vi "SimpleMotion2.vi"() -> ()   [LabVIEW 2019]
uses:
  Motion/EnableMultiple.vi
  Motion/MoveIncMultiple.vi
  Motion/WaitMultiple.vi
  Motion/DisableMultiple.vi
panel:
  out "Position 2":string
  in  "Distance 2":dbl=10000.0
  in  "Speed 2":dbl=5000.0
  in  "Axis Name 2":string="Y"
  out "Position":string
  in  "Distance":dbl=10000.0
  in  "Speed":dbl=5000.0
  in  "Axis Name":string="X"
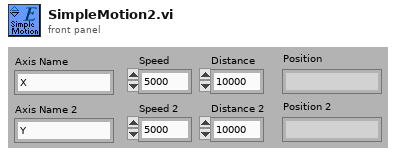
[diagram p1: front panel]
types:
  T1 = typedef "ControllerDiagPacket.ctl" = cluster{"Count":i32, "Packet Time":i64, "Axes":T2[], "error":errorcluster}
  T2 = typedef "AxisDiagPacket.ctl" = cluster{"Axis Name":string, "Acceleration Command":dbl, "Amplifier Temperature":sgl, "Analog Input 0":dbl, "Analog Input 1":dbl, "Analog Output 0":dbl, "Analog Output 1":dbl, "Axis Fault (num)":i32, "Axis Fault (str)":string, "Axis Fault (bits)":cluster{"AmplifierFault":bool, "AmplifierTemperatureFault":bool, "CcwEndOfTravelLimitFault":bool, "CcwSoftwareLimitFault":bool, "CommunicationLostFault":bool, "CwEndOfTravelLimitFault":bool, "CwSoftwareLimitFault":bool, "EmergencyStopFault":bool, "EncoderFault":bool, "ExternalFault":bool, "FeedbackScalingFault":bool, "HallSensorFault":bool, "MarkerSearchFault":bool, "MaxVelocityCommandFault":bool, "MotorTemperatureFault":bool, "None":bool, "OverCurrentFault":bool, "PositionErrorFault":bool, "PositionFeedbackFault":bool, "PowerSupplyFault":bool, "VelocityErrorFault":bool, "VelocityFeedbackFault":bool, "VoltageClampFault":bool}, "Axis Status (num)":i32, "Axis Status (str)":string, "Axis Status (bits)":cluster{"AccelerationPhase":bool, "AutofocusActive":bool, "BrakeOutput":bool, "CalibrationActive":bool, "CalibrationEnabled":bool, "CcwEndOfTravelLimitInput":bool, "CommandShapingFilterDone":bool, "CosineEncoderError":bool, "CurrentClamp":bool, "CwEndOfTravelLimitInput":bool, "DecelerationPhase":bool, "EmergencyStopInput":bool, "Enabled":bool, "GantryMasterActive":bool, "GantryModeActive":bool, "HallAInput":bool, "HallBInput":bool, "HallCInput":bool, "Homed":bool, "HomeLimitInput":bool, "Homing":bool, "InPosition":bool, "InPosition2":bool, "JoystickControl":bool, "MarkerInput":bool, "MasterMotionSuppressed":bool, "MasterSlaveControl":bool, "MotionIsCw":bool, "MoveActive":bool, "None":bool, "PositionCaptureActive":bool, "ServoControl":bool, "SineEncoderError":bool}, "Current Command":sgl, "Current Error":sgl, "Current Feedback":sgl, "Digital Input 0":i32, "Digital Input 1":i32, "Digital Input 2":i32, "Digital Output 0":i32, "Digital Output 1":i32, "Digital Output 2":i32, "Position Feedback Auxiliary":dbl, "Position Command":dbl, "Position Error":dbl, "Position Feedback":dbl, "Program Position Command":dbl, "Program Position Error":dbl, "Program Position Feedback":dbl, "Velocity Command":dbl, "Velocity Error":dbl, "Velocity Feedback":dbl}
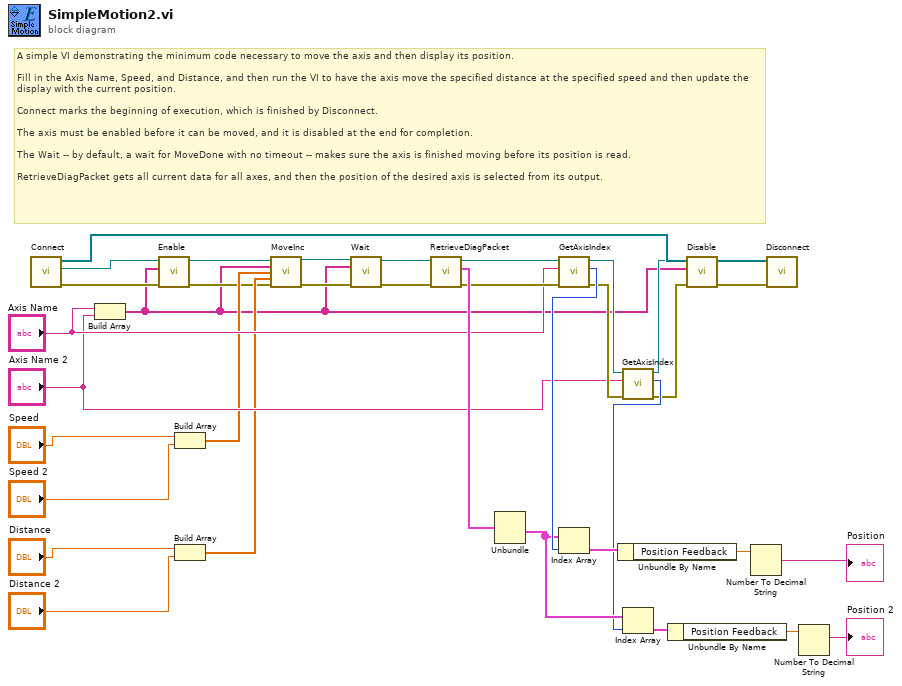
[diagram p0: block diagram]
diagram:
  # "A simple VI demonstrating the minimum code necessary to move the axis and then display its position.\n\nFill in the Axis Name, Speed, and Distance, and then run the VI to have the axis move the specified distance at the specified speed and then update the display with the current position.\n\nConnect marks the beginning of execution, which is finished by Disconnect.\n\nThe axis must be enabled before it can be moved, and it is disabled at the end for completion.\n\nThe Wait -- by default, a wait for MoveDone with no timeout -- makes sure the axis is finished moving before its position is read.\n\nRetrieveDiagPacket gets all current data for all axes, and then the position of the desired axis is selected from its output."
  n1 = call "Connect.vi"() -> ("error out"=w11:errorcluster, "controller"=w12:refnum<k24>, "controllers"=w31:refnum<k24>[])  [unwired: 9 in]
  n2 = Build Array("Axis Name", "Axis Name 2") -> (w3:string[])
  n3 = call-poly "Enable.vi"("error in (no error)"=w11, "axis names"=w3, "controller in"=w12) -> ("error out"=w10:errorcluster, "controller out"=w9:refnum<k24>)  [unwired: 7 in]
  n4 = Build Array("Speed", "Speed 2") -> (w14:dbl[])
  n5 = Build Array("Distance", "Distance 2") -> (w13:dbl[])
  n6 = call-poly "MoveInc.vi"("controller in"=w9, "axis names"=w3, "speeds"=w14, "distances"=w13, "error in (no error)"=w10) -> ("controller out"=w2:refnum<k24>, "error out"=w5:errorcluster)  [unwired: 9 in]
  n7 = call-poly "Wait.vi"("error in (no error)"=w5, "axis names"=w3, "controller in"=w2) -> ("error out"=w4:errorcluster, "controller out"=w1:refnum<k24>)  [unwired: 6 in, 1 out]
  n8 = call "RetrieveDiagPacket.vi"("error in (no error)"=w4, "Controller In"=w1) -> ("error out"=w33:errorcluster, "ControllerDiagPacket"=w35:T1, "Controller Out"=w21:refnum<k24>)  [unwired: 7 in]
  n9 = Unbundle(w35) -> ("Axes"=w25:T2[])  [unwired: 3 out]
  n10 = call "GetAxisIndex.vi"("error in (no error)"=w33, "axis name"="Axis Name", "controller in"=w21) -> ("error out"=w22:errorcluster, "axis index"=w32:i32, "controller out"=w7:refnum<k24>)  [unwired: 6 in]
  n11 = Index Array(array=w25, index=w32) -> (element=w30:T2)
  n12 = Unbundle By Name(w30) -> ("Position Feedback"=w29:dbl)
  n13 = call "GetAxisIndex.vi"("error in (no error)"=w22, "axis name"="Axis Name 2", "controller in"=w7) -> ("error out"=w23:errorcluster, "axis index"=w24:i32, "controller out"=w6:refnum<k24>)  [unwired: 6 in]
  n14 = Index Array(array=w25, index=w24) -> (element=w26:T2)
  n15 = Unbundle By Name(w26) -> ("Position Feedback"=w28:dbl)
  n16 = call-poly "Disable.vi"("error in (no error)"=w23, "axis names"=w3, "controller in"=w6) -> ("error out"=w8:errorcluster)  [unwired: 7 in, 1 out]
  n17 = Number To Decimal String(number=w29) -> (decimal integer string=→"Position":string)  [unwired: 1 in]
  n18 = call "Disconnect.vi"("error in (no error)"=w8, "controllers"=w31) -> ()  [unwired: 9 in, 1 out]
  n19 = Number To Decimal String(number=w28) -> (decimal integer string=→"Position 2":string)  [unwired: 1 in]
